vi "Validate Rate.vi"(8 "error IO":errorcluster, 10 "rate":dbl[unit] caption="Rate", 11 "Power Supply in":refnum<class "Power Supply.lvclass">) -> (0 "error out":errorcluster, 1 "Max rate":dbl[unit], 2 "Coerced rate":dbl[unit], 3 "Power Supply out":refnum<class "Power Supply.lvclass">, 4 "Coerced?":bool, 6 "Field":dbl[unit])   [LabVIEW 2023, in "Power Supply.lvclass"]
doc: "Query the current field and verify that the given sweep rate is appropriate for this field."
uses:
  Power Supply.lvclass
  Power Supply.lvclass/Power Supply.ctl
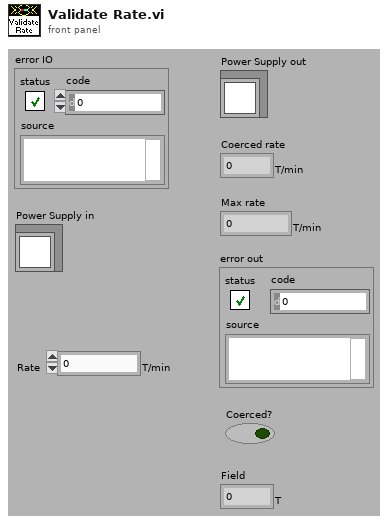
[diagram p1: front panel]
types:
  T1 = cluster{"Training Field":dbl[unit][], "Training Speed":dbl[unit][]}
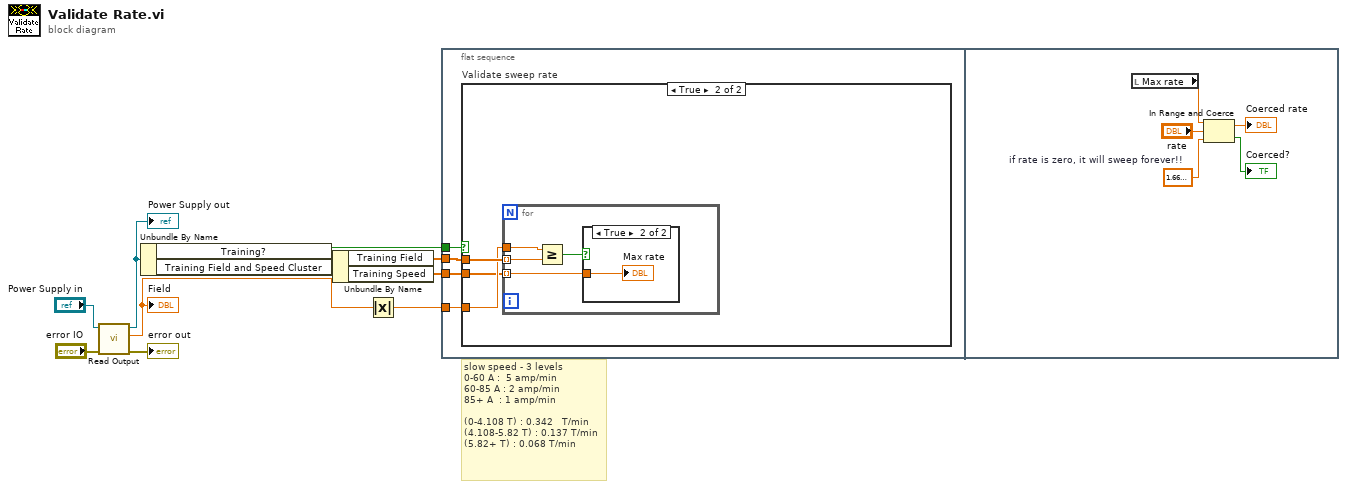
[diagram p0: block diagram]
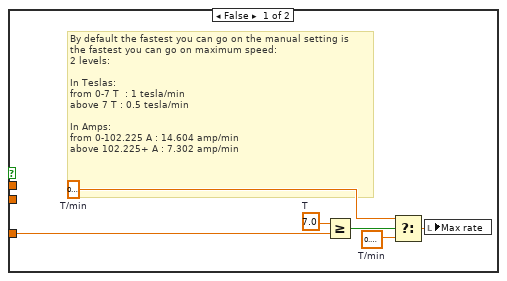
[diagram p2: hidden frame]
diagram:
  # "slow speed - 3 levels\n0-60 A :  5 amp/min\n60-85 A : 2 amp/min\n85+ A  : 1 amp/min\n\n(0-4.108 T) : 0.342   T/min\n(4.108-5.82 T) : 0.137 T/min\n(5.82+ T) : 0.068 T/min"
  n1 = call-dynamic "Read Output.vi"("error in (no error)"="error IO", "Power Supply in"="Power Supply in") -> ("error out"=→"error out":errorcluster, "Field"=w10:dbl[unit], "Power Supply out"=w1:refnum<class "Power Supply.lvclass">)  [unwired: 5 in, 2 out]
  "Field" <- w10
  "Power Supply out" <- w1
  n2 = Unbundle By Name(w1) -> ("Training?"=w5:bool, "Training Field and Speed Cluster"=w4:T1)
  n3 = Unbundle By Name(w4) -> ("Training Field"=w3:dbl[unit][], "Training Speed"=w2:dbl[unit][])
  n4 = Absolute Value(x=w10) -> (abs(x)=w6:dbl[unit])
  n5 = flat-sequence {
    tunnel: w6 -> [w14]
    tunnel: w5 -> [w13]
    tunnel: w3 -> [w12]
    tunnel: w2 -> [w11]
    frame #0 {
      n6 = case "Validate sweep rate" shown="True" w13 {
        tunnel: w14 -> [w16 w22]
        tunnel: w12 -> [_ w23]
        tunnel: w11 -> [_ w21]
        frame False {
          w18 = dbl[unit] 0.008333333333333333  # T/min
          w17 = dbl[unit] 0.016666666666666666  # T/min
          w19 = dbl[unit] 7.0  # T
          # "By default the fastest you can go on the manual setting is\nthe fastest you can go on maximum speed:\n2 levels:\n\nIn Teslas:\nfrom 0-7 T  : 1 tesla/min\nabove 7 T : 0.5 tesla/min\n\nIn Amps:\nfrom 0-102.225 A : 14.604 amp/min\nabove 102.225+ A : 7.302 amp/min"
          n7 = Greater Or Equal?(x=w19, y=w16) -> (x >= y?=w20:bool)
          n8 = Select(t=w17, s=w20, f=w18) -> (s? t:f=w15:dbl[unit])
          n9 = local write "Max rate"(w15) -> ()
        }
        frame True {
          n10 = for {
            tunnel: w23 -> [w27] mode=indexing
            tunnel: w22 -> [w26]
            tunnel: w21 -> [w24] mode=indexing
            n11 = Greater Or Equal?(x=w26, y=w27) -> (x >= y?=w25:bool)
            n12 = case shown="True" w25 {
              tunnel: w24 -> [_ w28]
              frame False {
              }
              frame True {
                "Max rate" <- w28
              }
            }
          }
        }
      }
    }
    frame #1 {
      w29 = dbl[unit] 1.6666666666666667e-08  # if rate is zero, it will sweep forever!!
      n13 = local read "Max rate"() -> (w33:dbl[unit])
      n14 = In Range and Coerce(upper limit=w33, x="rate", lower limit=w29) -> (coerced(x)=→"Coerced rate":dbl[unit], In Range?=→"Coerced?":bool)
    }
  }
